vi "Print.vi"(8 "Error In":errorcluster, 9 "Byte Count":u32=1024, 10 "Attribute":string, 11 "Kiethley 2602 In":refnum<visa-resource-name>) -> (0 "Error Out":errorcluster, 2 "Output":string, 3 "Keithley 2602 Out":refnum<visa-resource-name>)   [LabVIEW 2012, in "Keithley-2602.lvlib"]
uses:
  Keithley-2602.lvlib
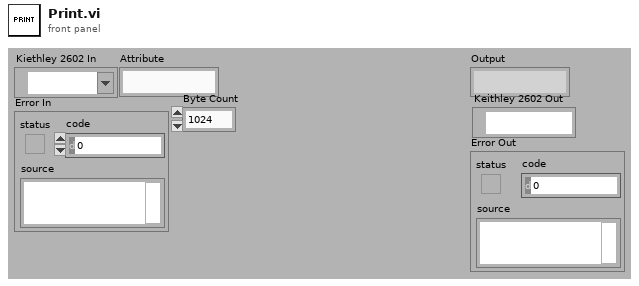
[diagram p1: front panel]
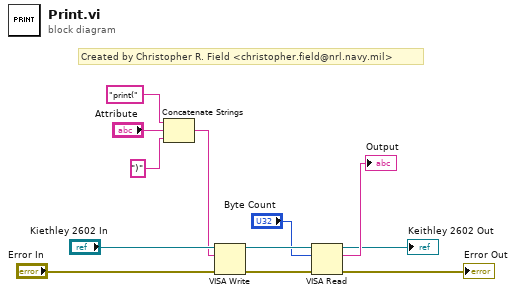
[diagram p0: block diagram]
diagram:
  # "Created by Christopher R. Field <christopher.field@nrl.navy.mil>"
  n1 = Concatenate Strings("print(", "Attribute", ")") -> (w7:string)
  n2 = VISA Write(VISA resource name="Kiethley 2602 In", write buffer=w7, error in (no error)="Error In") -> (VISA resource name out=w6:refnum<visa-resource-name>, error out=w5:errorcluster)  [unwired: 1 out]
  n3 = VISA Read(VISA resource name=w6, byte count="Byte Count", error in (no error)=w5) -> (VISA resource name out=→"Keithley 2602 Out":refnum<visa-resource-name>, read buffer=→"Output":string, error out=→"Error Out":errorcluster)  [unwired: 1 out]
